vi "ZDataVIS_Decimate+Fill_Intensity_Plot.vi"(7 "Voffset -2T":dbl, 8 "error in (no error)":errorcluster, 9 "fake point value":dbl, 10 "Decimate Controls":T1={"X Low"=-0.1, "X High"=0.1, "X Step"=4e-05, "Auto (T) or Manual (F) decimate"=FALSE, "auto steps"=0.0} {"X Step" format="%#_6p"; "X High" format="%#_6p"; "X Low" format="%#_6p"}, 11 "X and Y Arrays to decimate":T2(array[cluster])) -> (0 "error out":errorcluster, 1 "Offset X Low":dbl, 2 "Decimated X values":dbl[](array[numeric]), 3 "Arr of Y arrays (intensity info)":dbl[][](array[numeric]))   [LabVIEW 2016]
panel:
  out "Y size":i32
  out "X size":i32
  out "# y arrs":i32[](array[numeric])
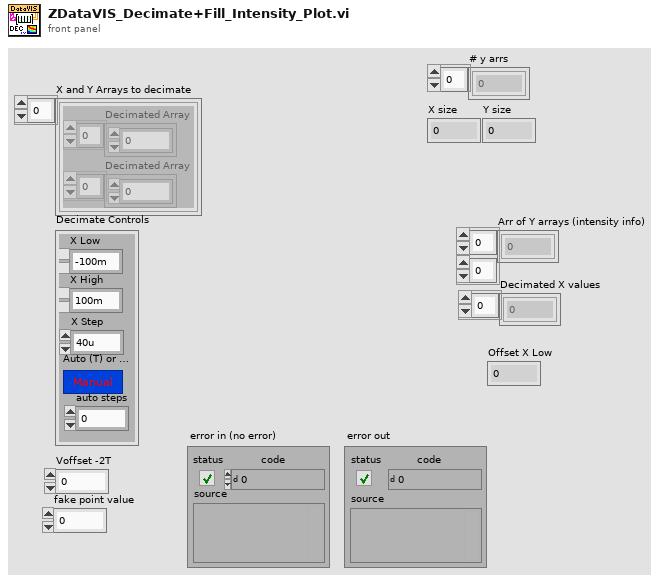
[diagram p1: front panel]
types:
  T1 = cluster{"X Low":dbl, "X High":dbl, "X Step":dbl, "Auto (T) or Manual (F) decimate":bool, "auto steps":dbl}
  T2 = cluster{"Decimated Array":dbl[], "Decimated Array":dbl[]}[]
  T3 = cluster{"Decimated Array":dbl[], "Decimated Array":dbl[]}
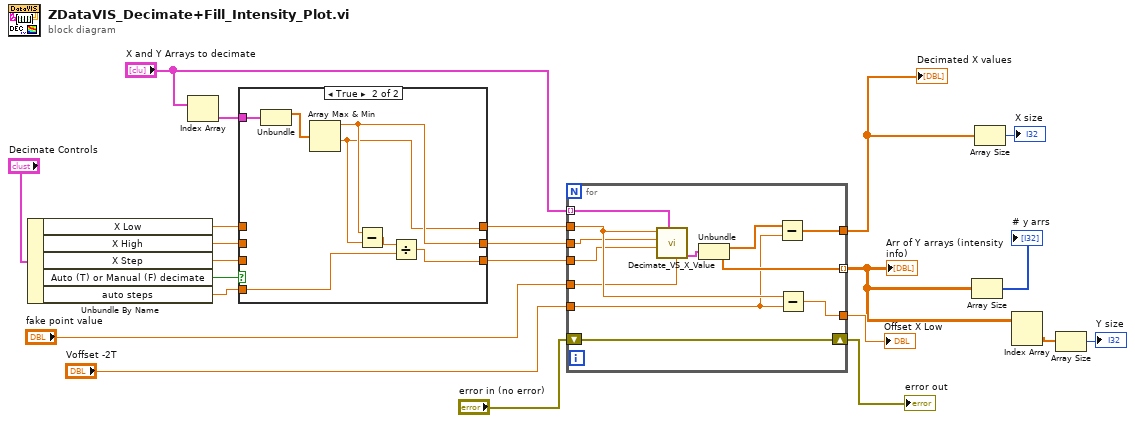
[diagram p0: block diagram]
diagram:
  n1 = Unbundle By Name("Decimate Controls") -> ("X Low"=w9:dbl, "X High"=w8:dbl, "X Step"=w7:dbl, "Auto (T) or Manual (F) decimate"=w10:bool, "auto steps"=w1:dbl)
  n2 = Index Array(array="X and Y Arrays to decimate") -> (element=w2:T3)  [unwired: 1 in]
  n3 = case shown="True" w10 {
    tunnel: w9 -> [w25 _]
    tunnel: w8 -> [w24 _]
    tunnel: w7 -> [w23 _]
    tunnel: [w25 w29] -> w6
    tunnel: [w24 w30] -> w5
    tunnel: [w23 w27] -> w4
    tunnel: w2 -> [_ w32]
    tunnel: w1 -> [_ w26]
    frame False {
    }
    frame True {
      n4 = Unbundle(w32) -> ("Decimated Array"=w31:dbl[])  [unwired: 1 out]
      n5 = Array Max & Min(array=w31) -> (max value=w30:dbl, min value=w29:dbl)  [unwired: 2 out]
      n6 = Subtract(x=w30, y=w29) -> (x-y=w28:dbl)
      n7 = Divide(x=w28, y=w26) -> (x/y=w27:dbl)
    }
  }
  n8 = for {
    tunnel: [w42] -> w20
    tunnel: [w43] -> w17
    tunnel: "X and Y Arrays to decimate" -> [w37] mode=indexing
    tunnel: [w41] -> w14 mode=indexing
    tunnel: w6 -> [w40]
    tunnel: w5 -> [w39]
    tunnel: w4 -> [w38]
    tunnel: "Voffset -2T" -> [w35]
    tunnel: "fake point value" -> [w34]
    shift-right: [w33] -> w18
    shift-left: "error in (no error)" -> [w33]
    n9 = call <userlib>:"Decimate_VS_X_Value.vi"("fake point value"=w34, "XY Graph kind 1"=w37, "X Step"=w38, "X High"=w39, "X Low"=w40) -> ("Interpolated"=w36:cluster{dbl[], dbl[]})  [unwired: 5 in, 1 out]
    n10 = Unbundle(w36) -> (w44:dbl[], w41:dbl[])
    n11 = Subtract(x=w44, y=w35) -> (x-y=w43:dbl[])
    n12 = Subtract(x=w40, y=w35) -> (x-y=w42:dbl)
  }
  "Decimated X values" <- w17
  "Arr of Y arrays (intensity info)" <- w14
  "Offset X Low" <- w20
  "error out" <- w18
  n13 = Array Size(array=w14) -> (size(s)=→"# y arrs":i32[])
  n14 = Array Size(array=w17) -> (size(s)=→"X size":i32)
  n15 = Index Array(array=w14) -> (element=w13:dbl[])  [unwired: 2 in]
  n16 = Array Size(array=w13) -> (size(s)=→"Y size":i32)
